vi "PD demodulation cRIO.vi"(8 "error out":errorcluster, 10 "Sample rate":dbl, 11 "queue out":refnum<queue>) -> ()   [LabVIEW 2021]
uses:
  <vilib>/Utility/file.llb/Write Delimited Spreadsheet (DBL).vi
panel:
  out "Num pts Neg 3":i32=64
  out "Demodulated signal 3":dbl(graph)
  out "Num pts Pos 3":i32=64
  out "Num pts Neg":i32=64
  out "Demodulated signal 1":dbl(graph)
  out "Modulation frequency":dbl=100.0
  out "Num pts Pos":i32=64
  out "Num pts Neg 2":i32=64
  out "Demodulated signal 2":dbl(graph)
  out "Num pts Pos 2":i32=64
  out "High level":bool=TRUE
  out "Low level":bool
  out "Normalized signal 1":dbl(graph)
  out "Normalized signal 2":dbl(graph)
  in  "Save data":bool caption="Enable"
  in  "Filename":path=path "C:/Users/data/2023_09_14_NI9230_pd-demodulation-12_8ks_100Hzmod_85mA_10c_ch1_demod1_ch2_demod2_ch3_demodpower_mid1_mid3_001.lvm"
  out "Arrays in queue":i32
  in  "Consumer loop update rate (ms)":u32=10
  out "Consumer loop time":u32=101
  out "Array size":i32
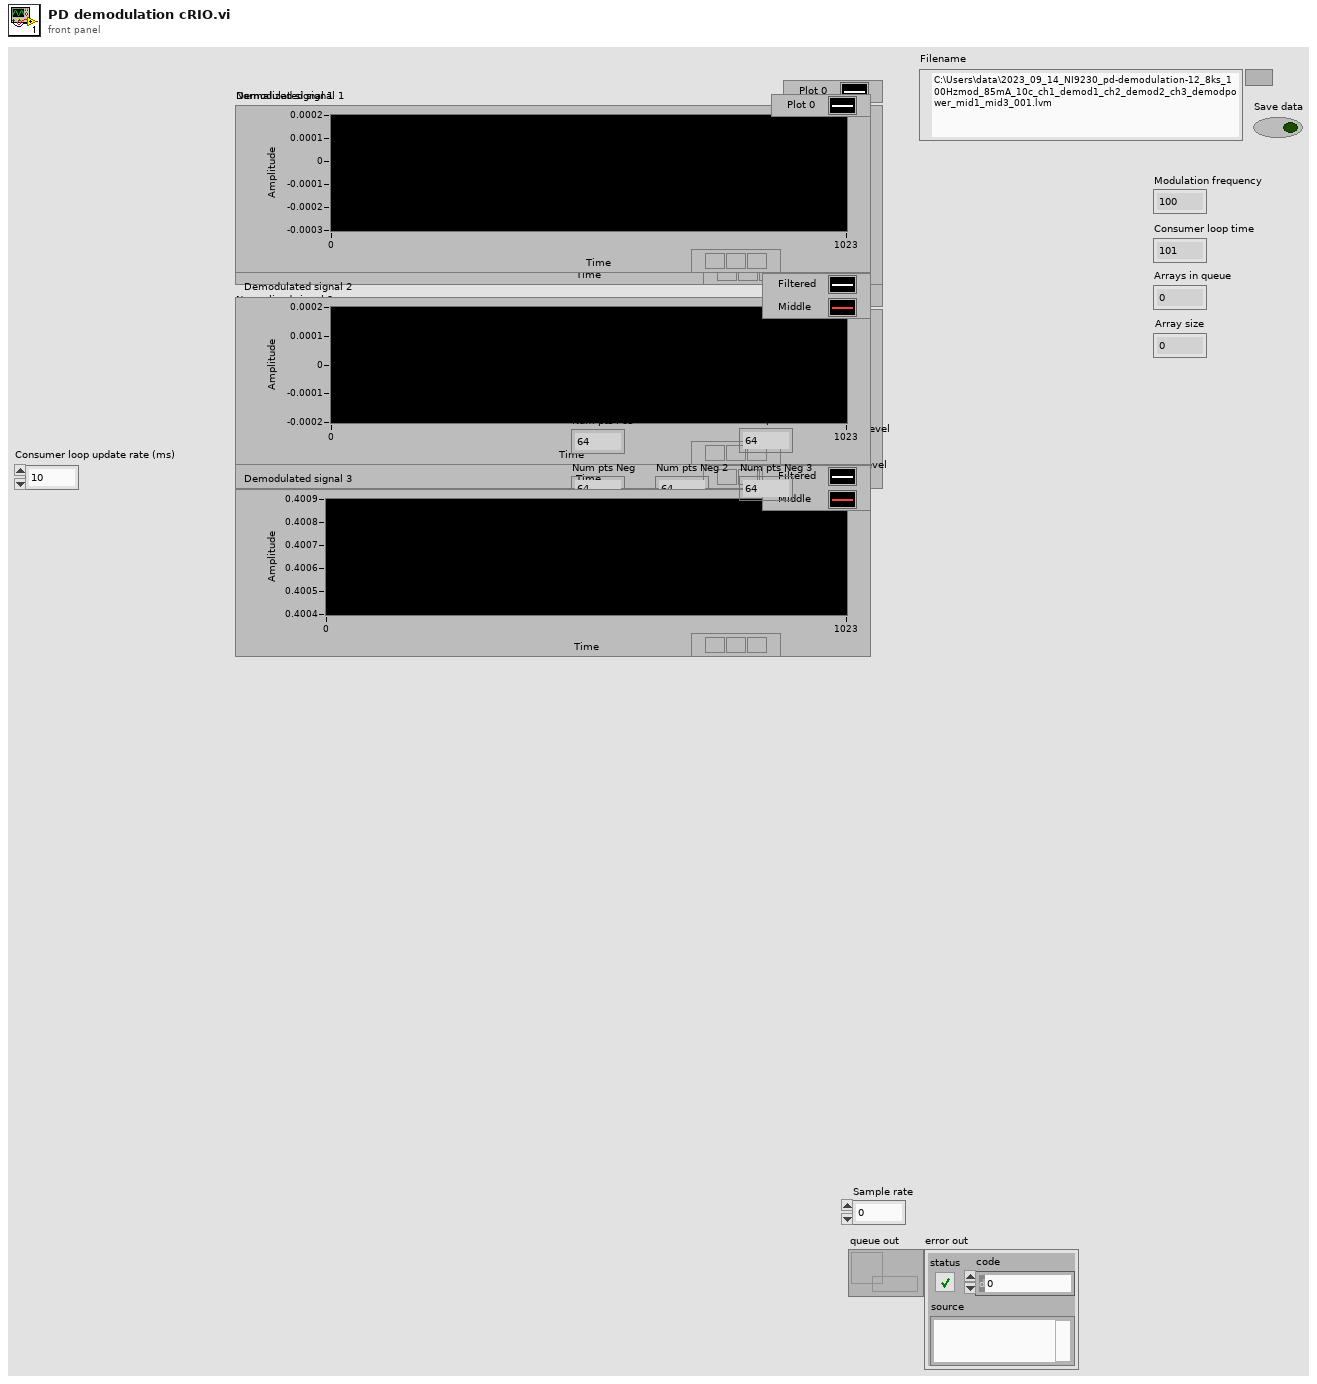
[diagram p1: front panel]
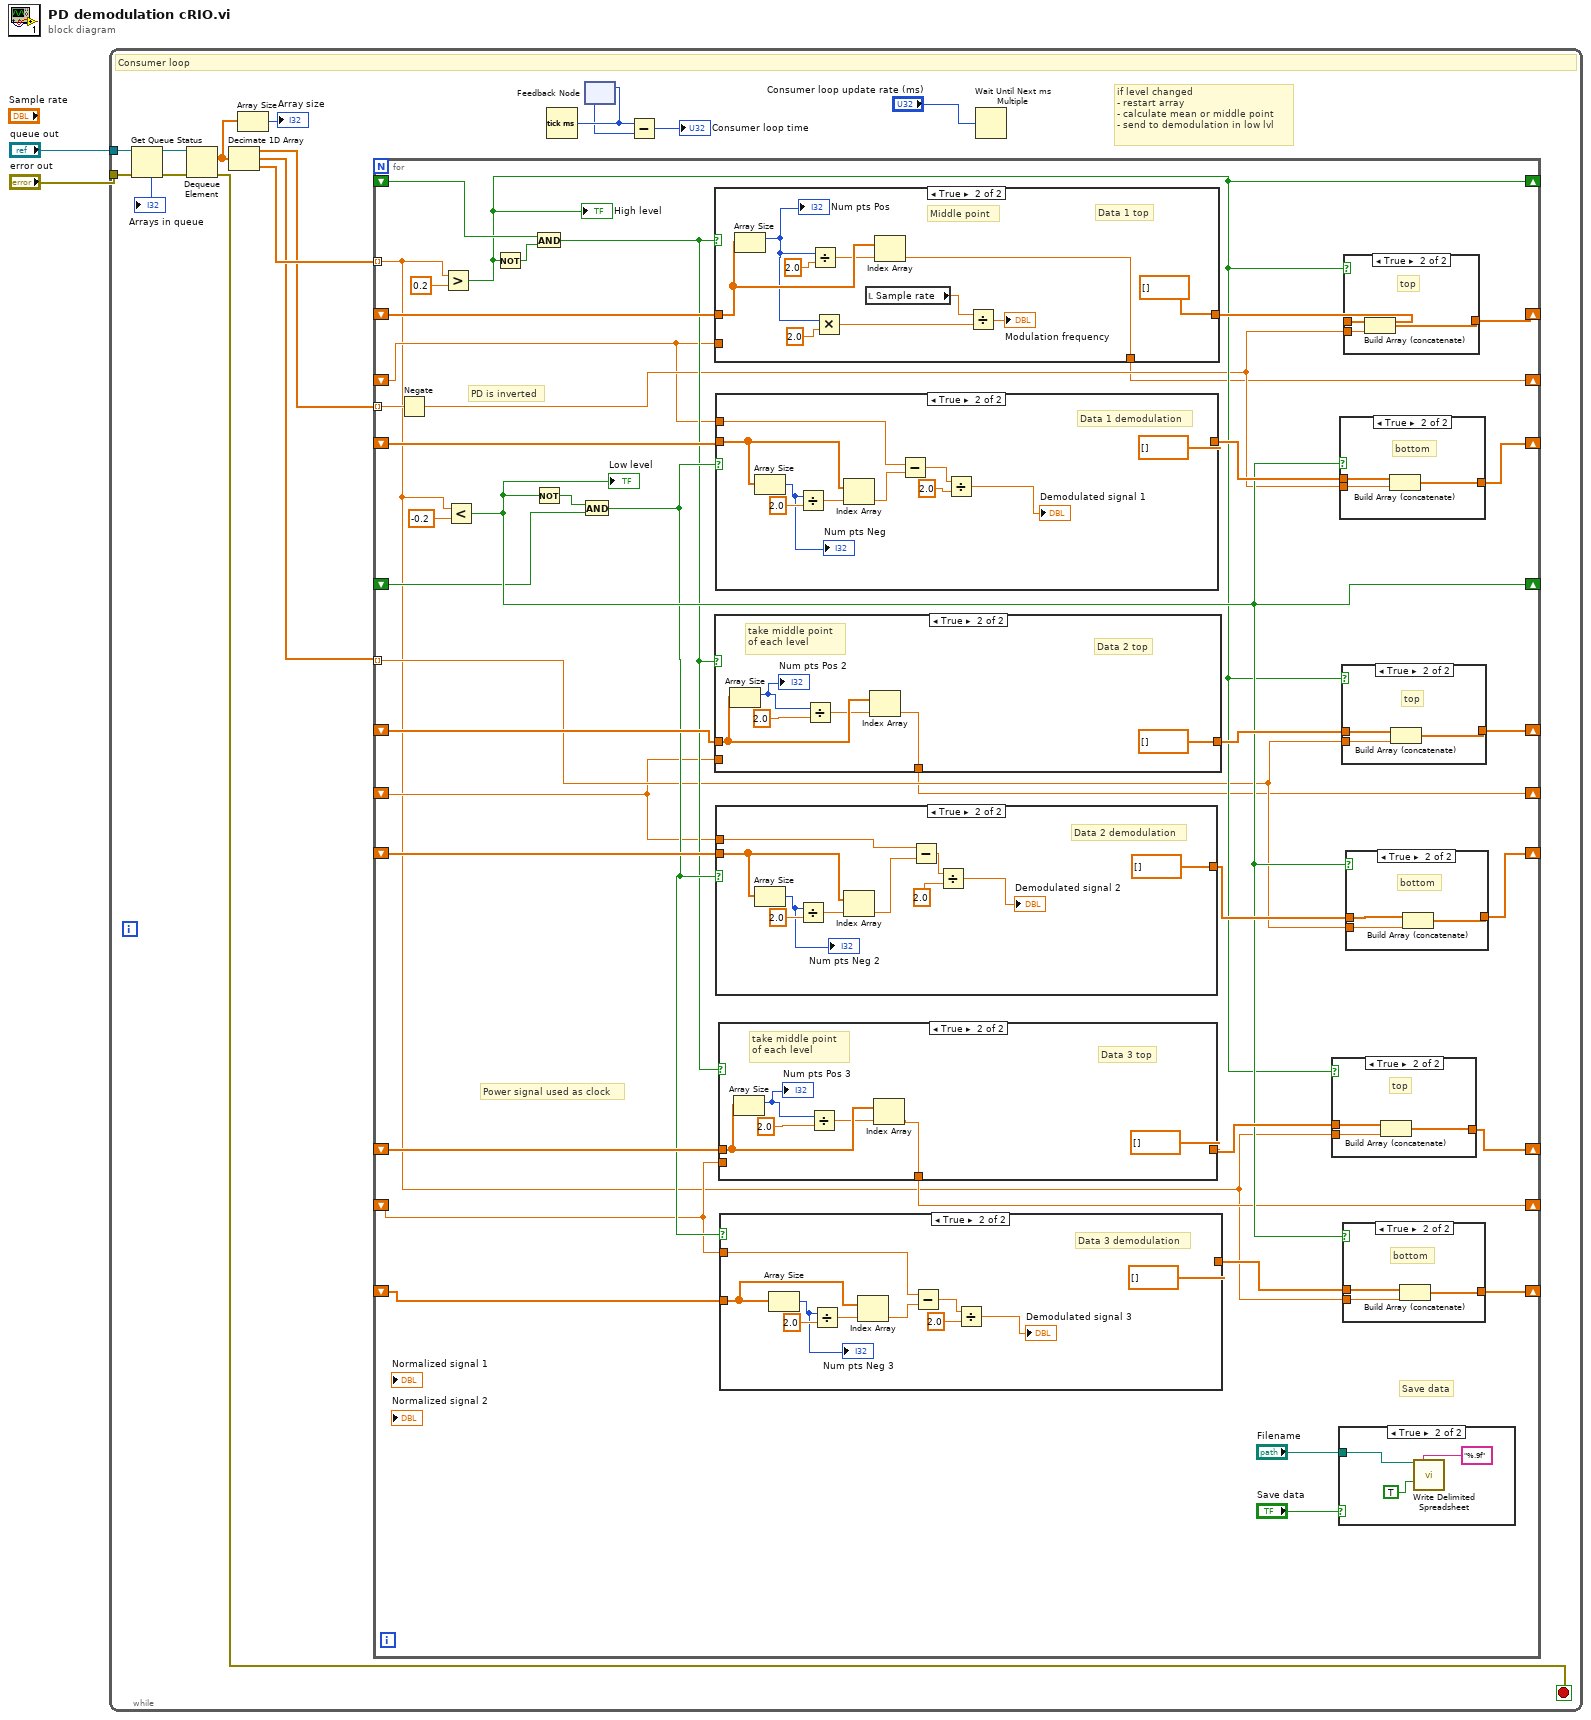
[diagram p0: block diagram]
diagram:
  n1 = while {
    tunnel: "queue out" -> [w13]
    tunnel: "error out" -> [w14]
    stop <- w15 stop-if-true
    # "if level changed\n- restart array\n- calculate mean or middle point\n- send to demodulation in low lvl"
    # "Consumer loop"
    n2 = Get Queue Status(queue=w13, error in (no error)=w14) -> (queue out=w12:refnum<queue>, error out=w11:errorcluster, # elements in queue=→"Arrays in queue":i32)  [unwired: 1 in, 5 out]
    n3 = Dequeue Element(queue=w12, error in (no error)=w11) -> (element=w10:dbl[], error out=w15:errorcluster)  [unwired: 1 in, 2 out]
    n4 = Decimate 1D Array(w10) -> (w5:dbl[], w6:dbl[], w7:dbl[])
    n5 = Array Size(array=w10) -> (size(s)=→"Array size":i32)
    n6 = for {
      tunnel: w7 -> [w18] mode=indexing
      shift-right: [w32] -> _
      shift-left: _ -> [w54]
      shift-right: [w35] -> _
      shift-left: _ -> [w28]
      shift-right: [w51] -> _
      shift-left: _ -> [w53]
      shift-right: [w52] -> _
      shift-left: _ -> [w48]
      tunnel: w5 -> [w31] mode=indexing
      tunnel: w6 -> [w25] mode=indexing
      shift-right: [w45] -> _
      shift-left: _ -> [w46]
      shift-right: [w44] -> _
      shift-left: _ -> [w42]
      shift-right: [w39] -> _
      shift-left: _ -> [w40]
      shift-right: [w37] -> _
      shift-left: _ -> [w36]
      shift-right: [w27] -> _
      shift-left: _ -> [w26]
      shift-right: [w24] -> _
      shift-left: _ -> [w21]
      shift-right: [w23] -> _
      shift-left: _ -> [w22]
      # "Save data"
      # "PD is inverted"
      # "Power signal used as clock"
      n7 = Negate(x=w31) -> (-x=w30:dbl)
      n8 = Greater?(x=w18, y=0.2) -> (0:w32:bool)
      "High level" <- w32
      n9 = Less?(x=w18, y=-0.2) -> (x < y?=w35:bool)
      "Low level" <- w35
      n10 = Not(x=w32) -> (.not. x?=w56:bool)
      n11 = And(x=w54, y=w56) -> (x .and. y?=w33:bool)
      n12 = Not(x=w35) -> (.not. x?=w29:bool)
      n13 = And(x=w29, y=w28) -> (x .and. y?=w34:bool)
      n14 = case shown="True" w33 {
        tunnel: [w81 dbl[] []] -> w49
        tunnel: w48 -> [w81 w88]
        tunnel: [w80 w84] -> w27
        tunnel: w26 -> [w80 _]
        frame False {
        }
        frame True {
          # "Middle point"
          # "Data 1 top"
          n15 = Array Size(array=w88) -> (size(s)=w87:i32)
          "Num pts Pos" <- w87
          n16 = Divide(x=w87, y=2.0) -> (x/y=w86:dbl)
          n17 = Multiply(x=w87, y=2.0) -> (x*y=w89:dbl)
          n18 = local read "Sample rate"() -> (w90:dbl)
          n19 = Index Array(array=w88, index=w86) -> (element=w84:dbl)
          n20 = Divide(x=w90, y=w89) -> (x/y=→"Modulation frequency":dbl)
        }
      }
      n21 = case shown="True" w33 {
        tunnel: [w62 dbl[] []] -> w47
        tunnel: w42 -> [w62 w66]
        tunnel: [w61 w63] -> w24
        tunnel: w21 -> [w61 _]
        frame False {
        }
        frame True {
          # "Data 2 top"
          # "take middle point \nof each level"
          n22 = Array Size(array=w66) -> (size(s)=w65:i32)
          "Num pts Pos 2" <- w65
          n23 = Divide(x=w65, y=2.0) -> (x/y=w64:dbl)
          n24 = Index Array(array=w66, index=w64) -> (element=w63:dbl)
        }
      }
      n25 = case shown="True" w34 {
        tunnel: [w92 dbl[] []] -> w50
        tunnel: w53 -> [w92 w95]
        tunnel: w26 -> [_ w94]
        frame False {
        }
        frame True {
          # "Data 1 demodulation"
          n26 = Array Size(array=w95) -> (size(s)=w97:i32)
          "Num pts Neg" <- w97
          n27 = Divide(x=w97, y=2.0) -> (x/y=w96:dbl)
          n28 = Index Array(array=w95, index=w96) -> (element=w99:dbl)
          n29 = Subtract(x=w94, y=w99) -> (x-y=w101:dbl)
          n30 = Divide(x=w101, y=2.0) -> (x/y=→"Demodulated signal 1":dbl)
        }
      }
      n31 = case shown="True" w34 {
        tunnel: [w69 dbl[] []] -> w43
        tunnel: w46 -> [w69 w72]
        tunnel: w21 -> [_ w71]
        frame False {
        }
        frame True {
          # "Data 2 demodulation"
          n32 = Array Size(array=w72) -> (size(s)=w74:i32)
          "Num pts Neg 2" <- w74
          n33 = Divide(x=w74, y=2.0) -> (x/y=w73:dbl)
          n34 = Index Array(array=w72, index=w73) -> (element=w76:dbl)
          n35 = Subtract(x=w71, y=w76) -> (x-y=w78:dbl)
          n36 = Divide(x=w78, y=2.0) -> (x/y=→"Demodulated signal 2":dbl)
        }
      }
      n37 = case shown="True" w33 {
        tunnel: [w104 dbl[] []] -> w41
        tunnel: w40 -> [w104 w108]
        tunnel: [w103 w105] -> w23
        tunnel: w22 -> [w103 _]
        frame False {
        }
        frame True {
          # "Data 3 top"
          # "take middle point \nof each level"
          n38 = Array Size(array=w108) -> (size(s)=w107:i32)
          "Num pts Pos 3" <- w107
          n39 = Divide(x=w107, y=2.0) -> (x/y=w106:dbl)
          n40 = Index Array(array=w108, index=w106) -> (element=w105:dbl)
        }
      }
      n41 = case shown="True" w34 {
        tunnel: [w111 dbl[] []] -> w38
        tunnel: w36 -> [w111 w114]
        tunnel: w22 -> [_ w113]
        frame False {
        }
        frame True {
          # "Data 3 demodulation"
          n42 = Array Size(array=w114) -> (size(s)=w116:i32)
          "Num pts Neg 3" <- w116
          n43 = Divide(x=w116, y=2.0) -> (x/y=w115:dbl)
          n44 = Index Array(array=w114, index=w115) -> (element=w118:dbl)
          n45 = Subtract(x=w113, y=w118) -> (x-y=w120:dbl)
          n46 = Divide(x=w120, y=2.0) -> (x/y=→"Demodulated signal 3":dbl)
        }
      }
      n47 = case shown="True" w32 {
        tunnel: w41 -> [w142 w145]
        tunnel: [w142 w143] -> w39
        tunnel: w18 -> [_ w144]
        frame False {
        }
        frame True {
          # "top"
          n48 = Build Array (concatenate)(w145, w144) -> (w143:dbl[])
        }
      }
      n49 = case shown="True" "Save data" {
        tunnel: "Filename" -> [_ w58]
        frame False {
        }
        frame True {
          n50 = call-poly <vilib>:"Write Delimited Spreadsheet.vi"("file path (dialog if empty)"=w58, "format (%.3f)"="%.9f", "append to file? (new file:F)"=TRUE) -> ()  [unwired: 11 in, 2 out]
        }
      }
      n51 = case shown="True" w35 {
        tunnel: w50 -> [w130 w133]
        tunnel: w30 -> [_ w132]
        tunnel: [w130 w131] -> w51
        frame False {
        }
        frame True {
          # "bottom"
          n52 = Build Array (concatenate)(w133, w132) -> (w131:dbl[])
        }
      }
      n53 = case shown="True" w32 {
        tunnel: w47 -> [w126 w129]
        tunnel: [w126 w127] -> w44
        tunnel: w25 -> [_ w128]
        frame False {
        }
        frame True {
          # "top"
          n54 = Build Array (concatenate)(w129, w128) -> (w127:dbl[])
        }
      }
      n55 = case shown="True" w35 {
        tunnel: w38 -> [w138 w141]
        tunnel: [w138 w139] -> w37
        tunnel: w18 -> [_ w140]
        frame False {
        }
        frame True {
          # "bottom"
          n56 = Build Array (concatenate)(w141, w140) -> (w139:dbl[])
        }
      }
      n57 = case shown="True" w32 {
        tunnel: w49 -> [w134 w137]
        tunnel: [w134 w135] -> w52
        tunnel: w30 -> [_ w136]
        frame False {
        }
        frame True {
          # "top"
          n58 = Build Array (concatenate)(w137, w136) -> (w135:dbl[])
        }
      }
      n59 = case shown="True" w35 {
        tunnel: w43 -> [w122 w125]
        tunnel: [w122 w123] -> w45
        tunnel: w25 -> [_ w124]
        frame False {
        }
        frame True {
          # "bottom"
          n60 = Build Array (concatenate)(w125, w124) -> (w123:dbl[])
        }
      }
    }
    n61 = Tick Count (ms)() -> (millisecond timer value=w4:u32)
    n62 = feedback #1() -> (w3:u32)  [unwired: 1 in]
    n63 = feedback-in #1(w4) -> ()
    n64 = Subtract(x=w4, y=w3) -> (x-y=→"Consumer loop time":u32)
    n65 = Wait Until Next ms Multiple(millisecond multiple="Consumer loop update rate (ms)") -> ()  [unwired: 1 out]
  }
